vi "Get StateChange 802.11 Standard.vi"(8 "error in (no error)":errorcluster, 11 "niDTS WLAN DUT in":refnum<class "niDTS WLAN Dut.lvclass">) -> (0 "error out":errorcluster, 2 "Changed":bool, 3 "niDTS WLAN DUT out":refnum<class "niDTS WLAN Dut.lvclass">)   [LabVIEW 2015, in "niDTS WLAN.lvlib" / "niDTS WLAN Dut.lvclass"]
uses:
  niDTS WLAN Dut.lvclass
  niDTS WLAN Dut Data/niDTS WLAN Dut Data.lvclass
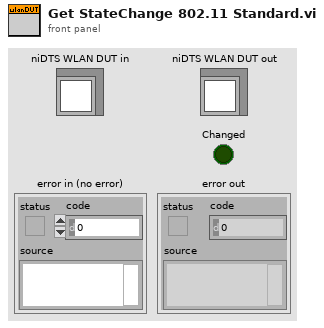
[diagram p1: front panel]
types:
  T1 = typedef "niDTS WLAN.lvlib/niDTS WLAN INC Standard.ctl" = enum16{"802.11 b DSSS", "802.11 a/g OFDM", "802.11 n HT", "802.11 ac VHT"}
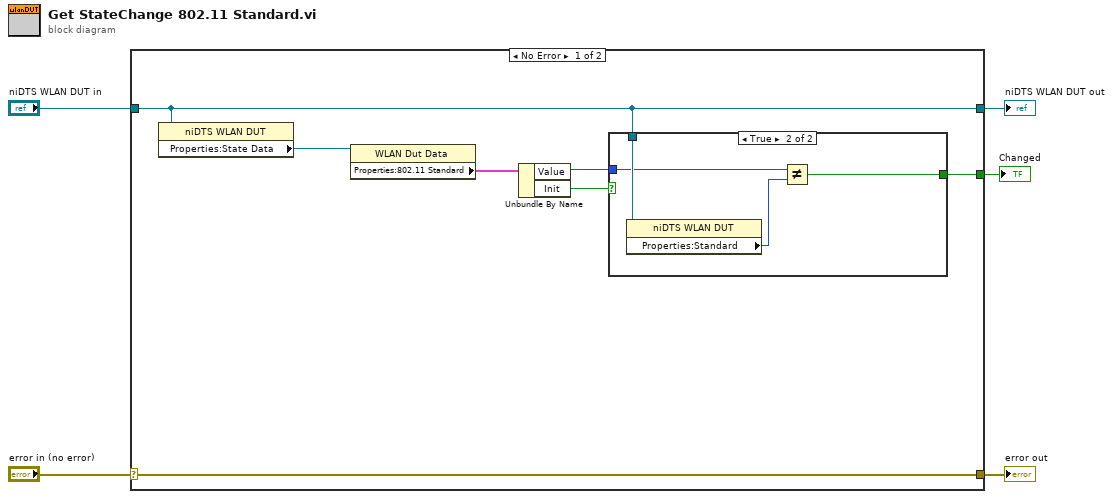
[diagram p0: block diagram]
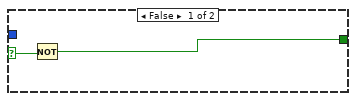
[diagram p2: hidden frame]
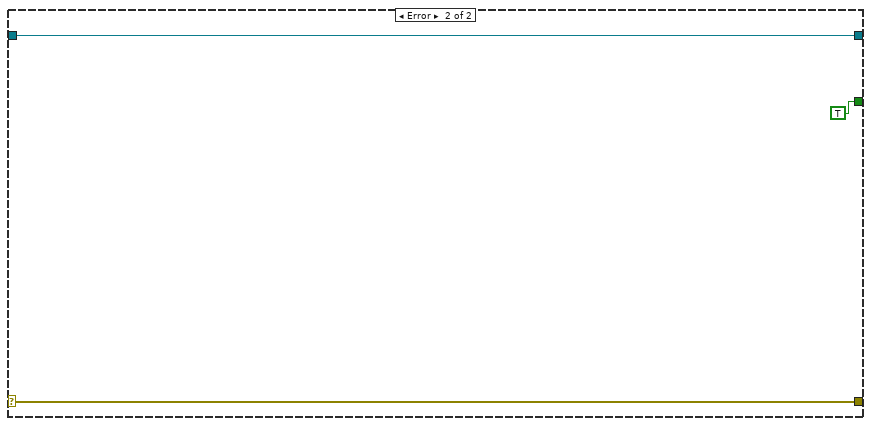
[diagram p3: hidden frame]
diagram:
  n1 = case shown="No Error" "error in (no error)" {
    selector: "error in (no error)" -> [w12 w21]
    tunnel: [w12 w21] -> w4
    tunnel: [w6 w20] -> w1
    tunnel: "niDTS WLAN DUT in" -> [w6 w20]
    tunnel: [w8 TRUE] -> w2
    frame No Error {
      n2 = property class="niDTS WLAN DUT"(reference=w6) -> ("Properties:State Data"=w11:refnum<class "niDTS WLAN Dut Data.lvclass">)  [unwired: 1 in, 2 out]
      n3 = property class="WLAN Dut Data"(reference=w11) -> ("Properties:802.11 Standard"=w10:cluster{"Value":T1, "Init":bool})  [unwired: 1 in, 2 out]
      n4 = Unbundle By Name(w10) -> ("Value"=w7:T1, "Init"=w9:bool)
      n5 = case shown="True" w9 {
        selector: w9 -> [w14 _]
        tunnel: [w13 w15] -> w8
        tunnel: w7 -> [_ w17]
        tunnel: w6 -> [_ w18]
        frame False {
          n6 = Not(x=w14) -> (.not. x?=w13:bool)
        }
        frame True {
          n7 = property class="niDTS WLAN DUT"(reference=w18) -> ("Properties:Standard"=w16:T1)  [unwired: 1 in, 2 out]
          n8 = Not Equal?(x=w17, y=w16) -> (x != y?=w15:bool)
        }
      }
    }
    frame Error {
    }
  }
  "error out" <- w4
  "niDTS WLAN DUT out" <- w1
  "Changed" <- w2
